vi "gRPC.HandleCancel.vi"(8 "error in (no error)":errorcluster, 11 "gRPCid in":T1) -> (0 "error out":errorcluster, 3 "Stop?":bool)   [LabVIEW 2025, in "bus_monitor_server_do.lvlib"]
uses:
  bus_monitor_server_do.lvlib
  <vilib>/gRPC/LabVIEW gRPC Library/Shared/grpcId.ctl
  <vilib>/gRPC/LabVIEW gRPC Library/grpc-lvsupport-release.lvlib
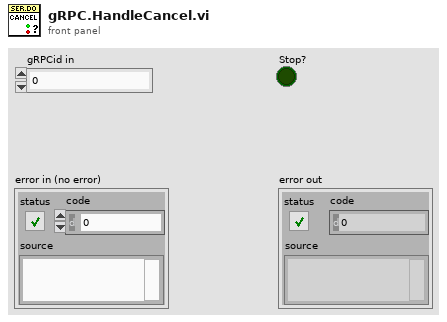
[diagram p1: front panel]
types:
  T1 = typedef "grpc-lvsupport-release.lvlib/grpcId.ctl" = u64
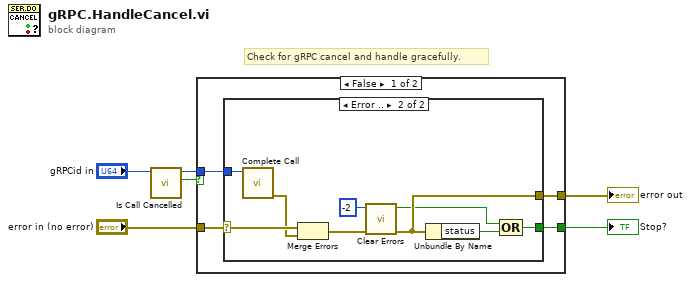
[diagram p0: block diagram]
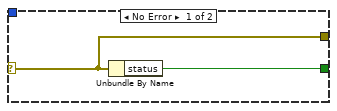
[diagram p2: hidden frame]
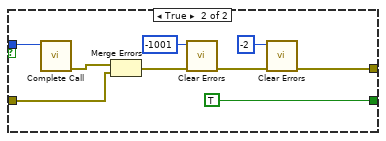
[diagram p3: hidden frame]
diagram:
  # "Check for gRPC cancel and handle gracefully."
  n1 = call <vilib>:"Is Call Cancelled.vi"("gRPCid in"="gRPCid in") -> ("Is Cancelled"=w2:bool, "gRPCid out"=w4:T1)  [unwired: 8 in, 1 out]
  n2 = case shown="False" w2 {
    tunnel: "error in (no error)" -> [w10 w26]
    tunnel: w4 -> [w9 w30]
    tunnel: [w8 TRUE] -> w5
    tunnel: [w7 w25] -> w6
    frame False {
      n3 = case shown="Error .." w10 {
        selector: w10 -> [w11 w20]
        tunnel: w9 -> [_ w21]
        tunnel: [w12 w15] -> w8
        tunnel: [w11 w16] -> w7
        frame No Error {
          n4 = Unbundle By Name(w11) -> ("status"=w12:bool)
        }
        frame Error {
          n5 = call <vilib>:"Complete Call.vi"("gRPCid"=w21) -> ("error out"=w19:errorcluster)  [unwired: 9 in]
          n6 = Merge Errors(w20, w19) -> (w13:errorcluster)
          n7 = call <vilib>:"Clear Errors.vi"("error in (no error)"=w13, "specific error code to clear (0: all)"=-2) -> ("error out"=w16:errorcluster, "specific error cleared?"=w14:bool)  [unwired: 4 in]
          n8 = Unbundle By Name(w16) -> ("status"=w18:bool)
          n9 = Compound Arithmetic op=OR(w14, w18) -> (w15:bool)
        }
      }
    }
    frame True {
      n10 = call <vilib>:"Complete Call.vi"("gRPCid"=w30) -> ("error out"=w28:errorcluster)  [unwired: 9 in]
      n11 = Merge Errors(w28, w26) -> (w23:errorcluster)
      n12 = call <vilib>:"Clear Errors.vi"("error in (no error)"=w23, "specific error code to clear (0: all)"=-1001) -> ("error out"=w22:errorcluster)  [unwired: 4 in, 1 out]
      n13 = call <vilib>:"Clear Errors.vi"("error in (no error)"=w22, "specific error code to clear (0: all)"=-2) -> ("error out"=w25:errorcluster)  [unwired: 4 in, 1 out]
    }
  }
  "error out" <- w6
  "Stop?" <- w5
